vi "lockinMON.vi"() -> ()   [LabVIEW 2011]
panel:
  out "SlideY":cluster{dbl, dbl}(slide)={0.0, -1.6336633663366336} scale=-1.0..1.0
  out "Slide 2":cluster{dbl, dbl}(slide)={0.0, -1.6336633663366336} scale=-1.0..1.0
  out "Y":dbl
  out "X":dbl
  in  "stop":bool
  in  "Lockin":refnum<visa-resource-name>
  in  "Sr 830 sensitivity":T1(ring)
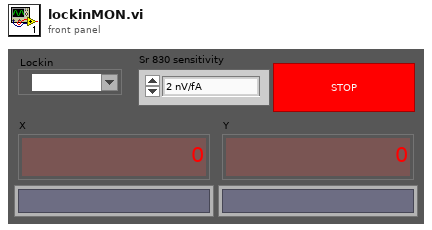
[diagram p1: front panel]
types:
  T1 = enum16{"2 nV/fA", "5 nV/fA", "10 nV/fA", "20 nV/fA", "50 nV/fA", "100 nV/fA", "200 nV/fA", "500 nV/fA", "1 uV/pA", "2 uV/pA", "5 uV/pA", "10 uV/pA", "20 uV/pA", "50 uV/pA", "100 uV/pA", "200 uV/pA", "500 uV/pA", "1 mV/nA", "2 mV/nA", "5 mV/nA", "10 mV/nA", "20 mV/nA", "50 mV/nA", "100 mV/nA", "200 mV/nA", "500 mV/nA", "1 V/uA"}
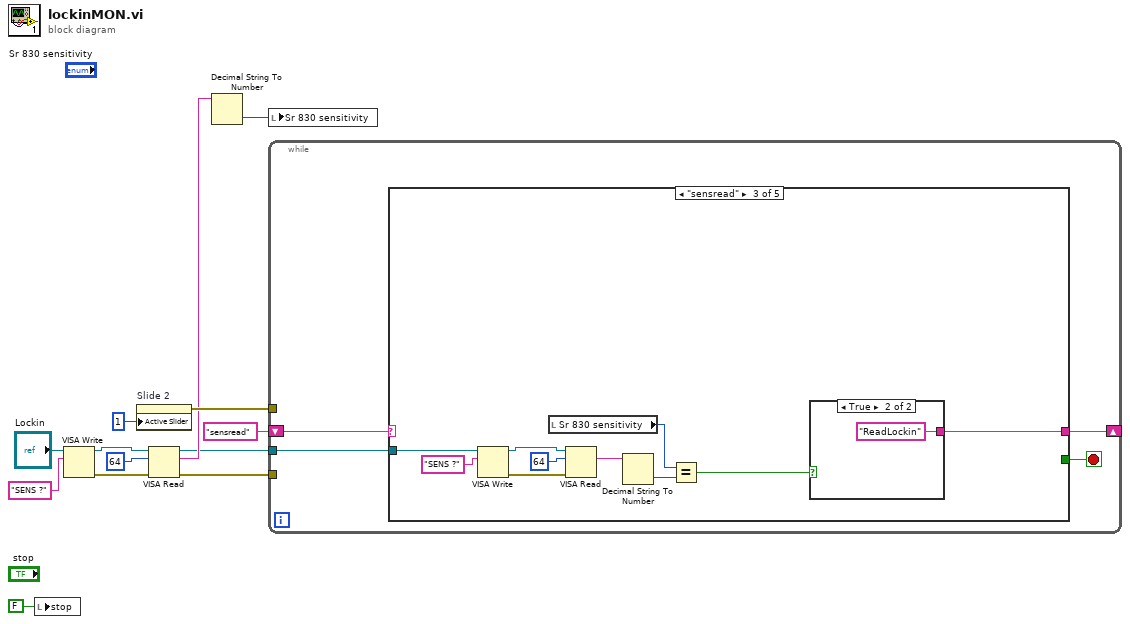
[diagram p0: block diagram]
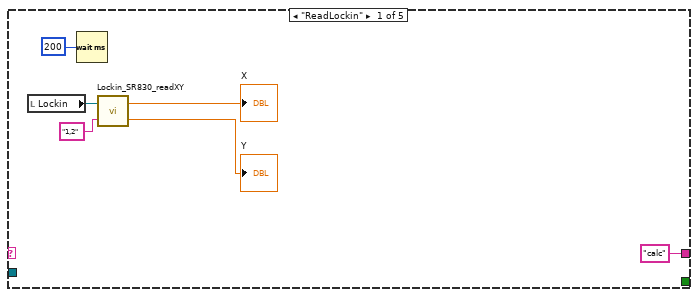
[diagram p2: hidden frame]
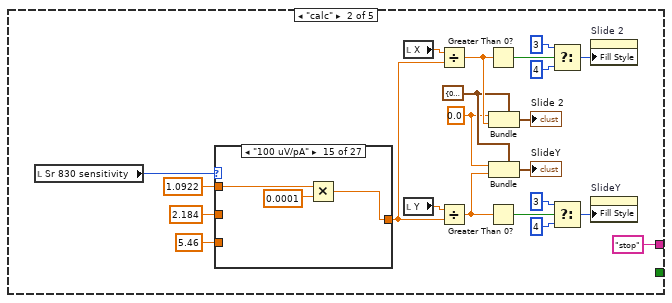
[diagram p3: hidden frame]
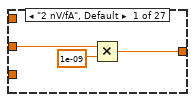
[diagram p4: hidden frame]
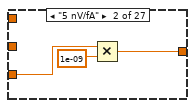
[diagram p5: hidden frame]
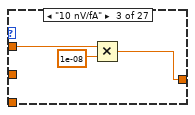
[diagram p6: hidden frame]
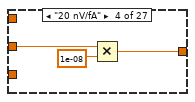
[diagram p7: hidden frame]
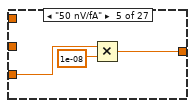
[diagram p8: hidden frame]
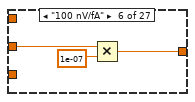
[diagram p9: hidden frame]
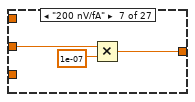
[diagram p10: hidden frame]
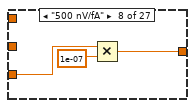
[diagram p11: hidden frame]
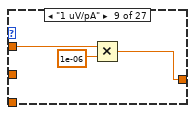
[diagram p12: hidden frame]
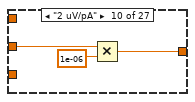
[diagram p13: hidden frame]
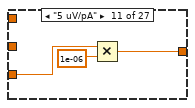
[diagram p14: hidden frame]
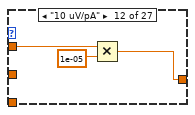
[diagram p15: hidden frame]
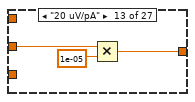
[diagram p16: hidden frame]
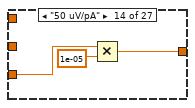
[diagram p17: hidden frame]
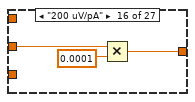
[diagram p18: hidden frame]
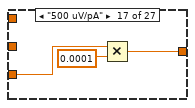
[diagram p19: hidden frame]
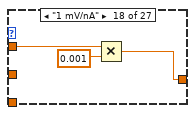
[diagram p20: hidden frame]
diagram:
  n1 = local write "stop"(FALSE ("stop")) -> ()
  n2 = VISA Write(VISA resource name="Lockin", write buffer="SENS ?" ("Command")) -> (VISA resource name out=w3:refnum<visa-resource-name>, error out=w6:errorcluster)  [unwired: 1 in, 1 out]
  n3 = property on="Slide 2" class="Slide (strict)"("Active Slider"=1) -> (error out=w11:errorcluster)  [unwired: 2 in, 1 out]
  n4 = VISA Read(VISA resource name=w3, byte count=u32 64 ("nombre d'octets"), error in (no error)=w6) -> (VISA resource name out=w1:refnum<visa-resource-name>, read buffer=w8:string, error out=w4:errorcluster)  [unwired: 1 out]
  n5 = Decimal String To Number(string=w8) -> (number=w9:i32)  [unwired: 2 in, 1 out]
  n6 = local write "Sr 830 sensitivity"(w9) -> ()
  n7 = while {
    shift-right: [w15] -> _
    shift-left: "sensread" -> [w17]
    tunnel: w1 -> [w14]
    tunnel: w11 -> [_]
    tunnel: w4 -> [_]
    stop <- w16 stop-if-true
    n8 = case shown="\"sensread\"" w17 {
      tunnel: [_ _ _ _ w144] -> w16
      tunnel: ["calc" "stop" w125 "ReadLockin" "sensread"] -> w15
      tunnel: w14 -> [_ _ w129 w138 _]
      frame "ReadLockin" {
        n9 = local read "Lockin"() -> (w23:refnum<visa-resource-name>)
        n10 = Wait (ms)(milliseconds to wait=u32 200) -> ()  [unwired: 1 out]
        n11 = call "Lockin_SR830_readXY.vi"("Variable"="1,2", "VISA Resource Name"=w23) -> ("Output Y"=→"Y":dbl, "Output X"=→"X":dbl)
      }
      frame "calc" {
        w31 = cluster{dbl, dbl} {0.0, 0.0} ("Slide")
        w29 = 0.0
        n12 = local read "Sr 830 sensitivity"() -> (w45:T1)
        n13 = case shown="\"100 uV/pA\"" w45 {
          tunnel: 1.0922 -> [_ _ w53 _ _ _ _ _ w71 _ _ w80 _ _ w89 _ _ w98 _ _ w107 _ _ w116 _ _ w124]
          tunnel: [w46 w49 w52 w55 w58 w61 w64 w67 w70 w73 w76 w79 w82 w85 w88 w91 w94 w97 w100 w103 w106 w109 w112 w115 w118 w121 w124] -> w39
          tunnel: 2.184 -> [w47 _ _ w56 _ w62 w65 _ _ w75 _ _ w83 _ _ w92 _ _ w101 _ _ w110 _ _ w119 _ _]
          tunnel: 5.46 -> [_ w50 _ _ w59 _ _ w68 _ _ w77 _ _ w86 _ _ w95 _ _ w104 _ _ w113 _ _ w122 _]
          frame "2 nV/fA", Default {
            n14 = Multiply(x=w47, y=1e-09) -> (x*y=w46:dbl)
          }
          frame "5 nV/fA" {
            n15 = Multiply(x=w50, y=1e-09) -> (x*y=w49:dbl)
          }
          frame "10 nV/fA" {
            n16 = Multiply(x=w53, y=1e-08) -> (x*y=w52:dbl)
          }
          frame "20 nV/fA" {
            n17 = Multiply(x=w56, y=1e-08) -> (x*y=w55:dbl)
          }
          frame "50 nV/fA" {
            n18 = Multiply(x=w59, y=1e-08) -> (x*y=w58:dbl)
          }
          frame "100 nV/fA" {
            n19 = Multiply(x=w62, y=1e-07) -> (x*y=w61:dbl)
          }
          frame "200 nV/fA" {
            n20 = Multiply(x=w65, y=1e-07) -> (x*y=w64:dbl)
          }
          frame "500 nV/fA" {
            n21 = Multiply(x=w68, y=1e-07) -> (x*y=w67:dbl)
          }
          frame "1 uV/pA" {
            n22 = Multiply(x=w71, y=1e-06) -> (x*y=w70:dbl)
          }
          frame "2 uV/pA" {
            n23 = Multiply(x=w75, y=1e-06) -> (x*y=w73:dbl)
          }
          frame "5 uV/pA" {
            n24 = Multiply(x=w77, y=1e-06) -> (x*y=w76:dbl)
          }
          frame "10 uV/pA" {
            n25 = Multiply(x=w80, y=1e-05) -> (x*y=w79:dbl)
          }
          frame "20 uV/pA" {
            n26 = Multiply(x=w83, y=1e-05) -> (x*y=w82:dbl)
          }
          frame "50 uV/pA" {
            n27 = Multiply(x=w86, y=1e-05) -> (x*y=w85:dbl)
          }
          frame "100 uV/pA" {
            n28 = Multiply(x=w89, y=0.0001) -> (x*y=w88:dbl)
          }
          frame "200 uV/pA" {
            n29 = Multiply(x=w92, y=0.0001) -> (x*y=w91:dbl)
          }
          frame "500 uV/pA" {
            n30 = Multiply(x=w95, y=0.0001) -> (x*y=w94:dbl)
          }
          frame "1 mV/nA" {
            n31 = Multiply(x=w98, y=0.001) -> (x*y=w97:dbl)
          }
          frame "2 mV/nA" {
            n32 = Multiply(x=w101, y=0.001) -> (x*y=w100:dbl)
          }
          frame "5 mV/nA" {
            n33 = Multiply(x=w104, y=0.001) -> (x*y=w103:dbl)
          }
          frame "10 mV/nA" {
            n34 = Multiply(x=w107, y=0.01) -> (x*y=w106:dbl)
          }
          frame "20 mV/nA" {
            n35 = Multiply(x=w110, y=0.01) -> (x*y=w109:dbl)
          }
          frame "50 mV/nA" {
            n36 = Multiply(x=w113, y=0.01) -> (x*y=w112:dbl)
          }
          frame "100 mV/nA" {
            n37 = Multiply(x=w116, y=0.1) -> (x*y=w115:dbl)
          }
          frame "200 mV/nA" {
            n38 = Multiply(x=w119, y=0.1) -> (x*y=w118:dbl)
          }
          frame "500 mV/nA" {
            n39 = Multiply(x=w122, y=0.1) -> (x*y=w121:dbl)
          }
          frame "1 V/uA" {
          }
        }
        n40 = local read "X"() -> (w41:dbl)
        n41 = local read "Y"() -> (w40:dbl)
        n42 = Divide(x=w41, y=w39) -> (x/y=w34:dbl)
        n43 = Divide(x=w40, y=w39) -> (x/y=w25:dbl)
        n44 = Greater Than 0?(x=w34) -> (x > 0?=w37:bool)
        n45 = Greater Than 0?(x=w25) -> (x > 0?=w28:bool)
        n46 = Bundle(cluster=w31, w29, w34) -> (→"Slide 2":cluster{dbl, dbl})
        n47 = Bundle(cluster=w31, w29, w25) -> (→"SlideY":cluster{dbl, dbl})
        n48 = Select(t=3 ("Fill Style"), s=w37, f=4 ("Fill Style")) -> (s? t:f=w32:i32)
        n49 = Select(t=3 ("Fill Style"), s=w28, f=4 ("Fill Style")) -> (s? t:f=w24:i32)
        n50 = property on="Slide 2" class="Slide (strict)"("Fill Style"=w32) -> ()  [unwired: 2 in, 2 out]
        n51 = property on="SlideY" class="Slide (strict)"("Fill Style"=w24) -> ()  [unwired: 2 in, 2 out]
      }
      frame "sensread" {
        n52 = VISA Write(VISA resource name=w129, write buffer="SENS ?" ("Command")) -> (VISA resource name out=w133:refnum<visa-resource-name>, error out=w132:errorcluster)  [unwired: 1 in, 1 out]
        n53 = local read "Sr 830 sensitivity"() -> (w127:T1)
        n54 = VISA Read(VISA resource name=w133, byte count=u32 64 ("nombre d'octets"), error in (no error)=w132) -> (read buffer=w130:string)  [unwired: 3 out]
        n55 = Decimal String To Number(string=w130) -> (number=w128:i32)  [unwired: 2 in, 1 out]
        n56 = Equal?(x=w127, y=w128) -> (x = y?=w126:bool)
        n57 = case shown="True" w126 {
          tunnel: ["senschange" "ReadLockin"] -> w125
          frame False {
          }
          frame True {
          }
        }
      }
      frame "senschange" {
        n58 = local read "Sr 830 sensitivity"() -> (w137:T1)
        n59 = Number To Decimal String(number=w137) -> (decimal integer string=w141:string)  [unwired: 1 in]
        n60 = Concatenate Strings("SENS " ("chaîne"), w141) -> (w139:string)
        n61 = VISA Write(VISA resource name=w138, write buffer=w139) -> ()  [unwired: 1 in, 3 out]
      }
      frame "stop", Default {
        n62 = local read "stop"() -> (w144:bool)
      }
    }
  }
